vi "RT9031prueba.vi"() -> ()   [LabVIEW 2020]
uses:
  <vilib>/Model Interface Toolkit/Model Interface Toolkit.lvclass
  <vilib>/Platform/TimedLoop/XDataNode/timing_clust.ctl
  <vilib>/Platform/TimedLoop/XDataNode/nitl_modes.ctl
  <vilib>/Platform/TimedLoop/XDataNode/wakeup.ctl
  <vilib>/Model Interface Toolkit/Model Interface Toolkit.lvclass/Model Interface Toolkit.ctl
  <vilib>/Model Interface Toolkit/Model Update.vi
  <vilib>/Model Interface Toolkit/Tick Model.vi
  <vilib>/Model Interface Toolkit/Probe Signals.vi
  <vilib>/Model Interface Toolkit/Multirate/Dispatch Model Tasks.vi
  <vilib>/Model Interface Toolkit/Call Model Start Routine.vi
  <vilib>/Model Interface Toolkit/Handle Error.vi
  <vilib>/Model Interface Toolkit/Multirate/Wait on Tasks.vi
  <vilib>/FPGAPlugInAG/cRIO-9031/niLvFpga_Open_cRIO-9031.vi
  <vilib>/rvi/interface/common/dynamic/niFpgaDynamicAddResources.vi
  <vilib>/Utility/error.llb/Error Cluster From Error Code.vi
  <vilib>/rvi/errors/niLvFpgaAdjustHostInterfaceError.vi
  <vilib>/Model Interface Toolkit/Check Error.vi
  <vilib>/Model Interface Toolkit/Generate Error Cluster.vi
  <vilib>/Platform/TimedLoop/scheduler/LVUserAPI/Fire Software-Triggered Timing Source.vi
  <vilib>/FPGAPlugInAG/Dynamic/niLvFpga_Close_Dynamic.vi
  <vilib>/Platform/TimedLoop/XDataNode/XDataNode.xnode
  <vilib>/rvi/interface/nirviOpenFPGA/nirviOpenFPGA.xnode
  FPGA Bitfiles/dqmhemuladordege_FPGATarget_MainFPGA_ARUjFlg7-es.lvbitx
  FPGA/Main FPGA.vi
  <vilib>/rvi/interface/nirviReadWriteControl/nirviReadWriteControl.xnode
  <vilib>/rvi/interface/nirviCloseFPGA/nirviCloseFPGA.xnode
  <vilib>/Platform/TimedLoop/XDataNode/XDNodeRunTimeDep.lvlib
  NiFpgaLv.dll
  <vilib>/rvi/interface/Simulation/niFpgaSimulationCallBeginRW.vi
panel:
  in  "IFPGA 2":dbl
  in  "SOC 2":dbl
  in  "Igen 2":dbl
  in  "Vbat 2":dbl
  in  "Vgen 2":dbl
  in  "debug":bool
  out "FPGA":refnum<k20>
  out "SOC inicial [HMI]":dbl
  out "T. Bateria [HMI]":dbl
  out "I Load [HMI]":dbl
  out "Iexc":dbl(graph)
  out "Relé encendido":bool
  in  "Debug Iexc":bool
  in  "Iexc [Debug]":dbl
  in  "Modulacion Corrientes [Debug]":dbl
  in  "Debug Corrientes":bool
  in  "Modulacion T001 y T002 [Debug]":dbl
  in  "Debug Voltajes":bool
  out "stop!":i16
  out "0, 1":i16
  out "Estado de Carga":dbl(graph)
  out "Corriente Generador":dbl(graph)
  out "Voltaje Generador":dbl(graph)
  in  "wm(rpm)":dbl=1500.0
  out "Falla W4":bool
  out "Falla W3":bool
  out "Falla W2":bool
  out "Falla W1":bool
  out "Falla U4":bool
  out "Falla U3":bool
  out "Falla U2":bool
  out "Falla U1":bool
  out "Falla T002":bool
  out "Falla T001":bool
  out "Propulsion":bool
  out "CLC":bool
  out "ON/OFF":bool
  out "IFPGA":dbl
  out "Simulation Time (s)":dbl
  out "Iteration Duration":i64
  out "error out 2":errorcluster
  out "error out":errorcluster
  out "Finished Late? [i-1]":bool
  in  "stop FPGA":bool
  out "ExcFPGA":fxp<+/-,20,5>
  out "Igen":dbl
  out "Tbat":dbl
  out "IBat":dbl
  out "SOC":dbl
  out "Vbat":dbl
  out "Vgen":dbl
  out "Error2":errorcluster
  out "Model2":refnum<class "Model Interface Toolkit.lvclass">
  out "Error":errorcluster
  out "Model":refnum<class "Model Interface Toolkit.lvclass">
  in  "Relaunch Model/FPGA":bool
  in  "Prepare to Stop execution":bool
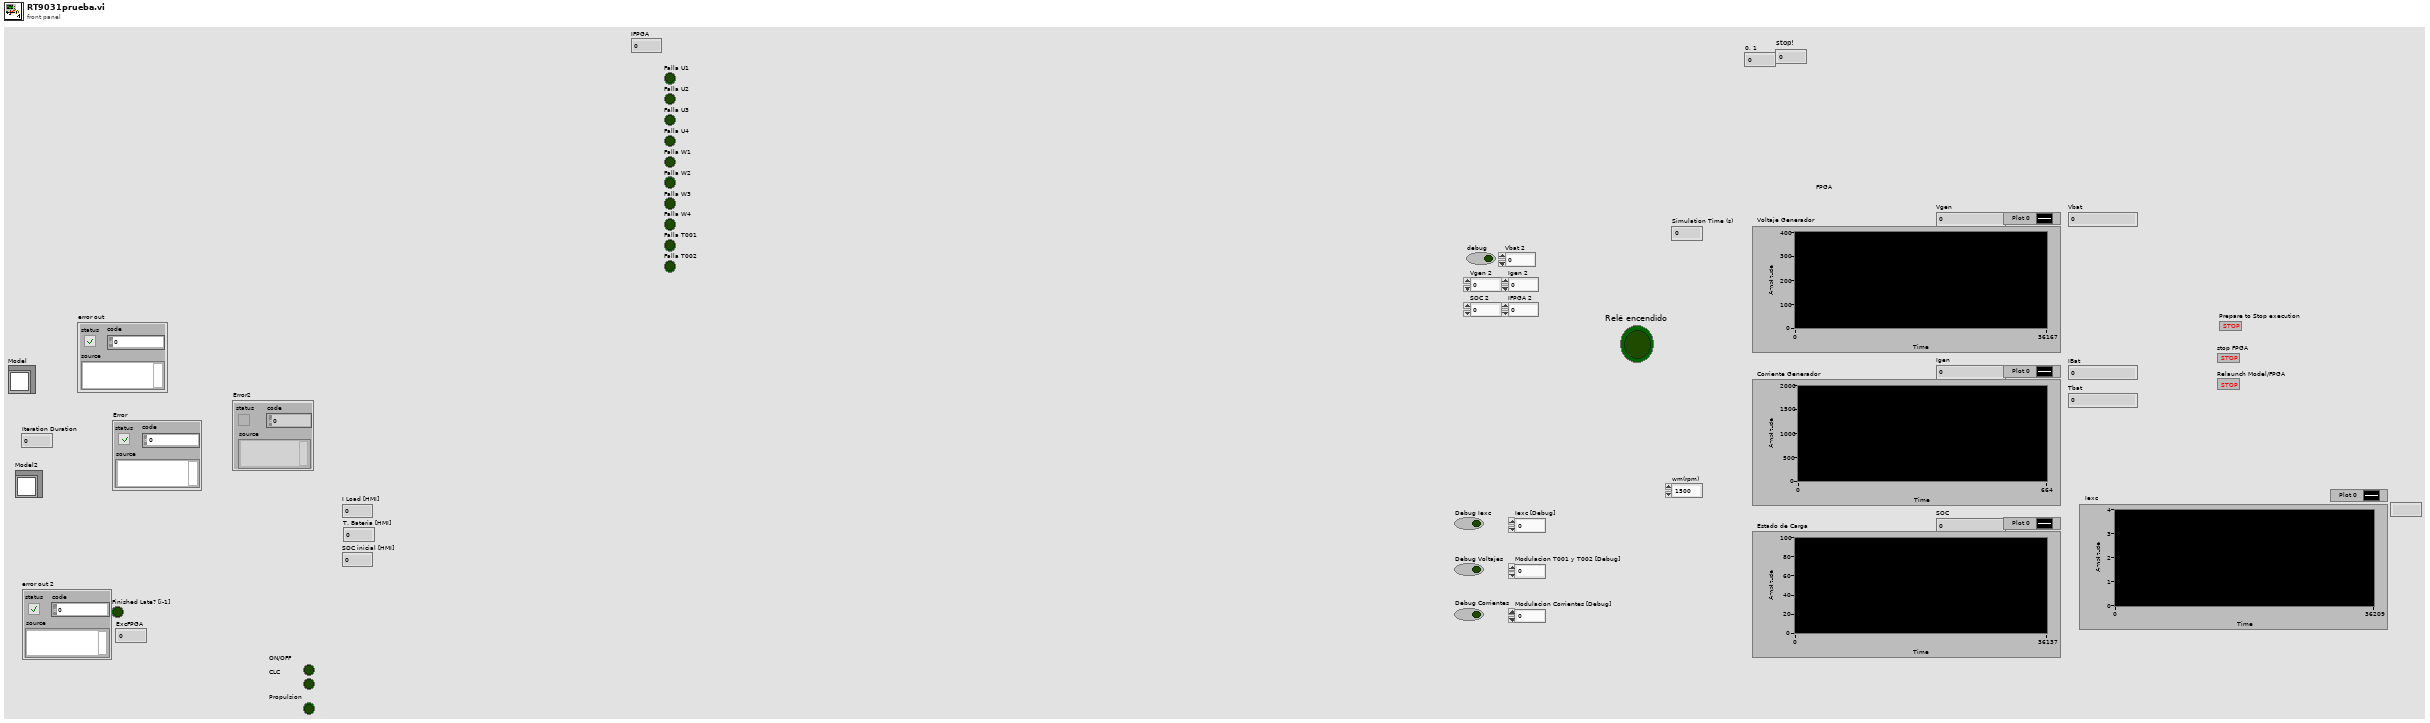
[diagram p1: front panel]
types:
  T1 = typedef "XDNodeRunTimeDep.lvlib/timing_clust.ctl" = cluster{"Expected End [f-1]":u64, "Actual End [f-1]":u64, "Finished Late? [f-1]":bool, "Expected End [i-1]":u64, "Actual End [i-1]":u64, "Finished Late? [i-1]":bool, "Expected Start [i]":u64, "Actual Start [i]":u64, "Expected Start [f]":u64, "Actual Start [f]":u64, "Source Name":string, "Structure Name":string, "Period":i64, "Deadline":i64, "Offset":i64, "Start":i64, "Priority":i32, "Timeout":i32, "Mode":T2, "Wakeup Reason":T3, "Error":errorcluster, "Source Type":string, "Secondary Source Type":string, "Global End Time":u64, "Global Start Time":u64, "Frame Duration":u64, "Iteration Duration":u64, "Assigned CPU":i32, "I/O Scan Engine Mode":u32}
  T2 = typedef "XDNodeRunTimeDep.lvlib/nitl_modes.ctl" = enum32{"No Change", "Process missed periods, maintain original phase", "Discard missed periods, maintain original phase", "Process missed periods, ignore original phase", "Discard missed periods, ignore original phase"}
  T3 = typedef "XDNodeRunTimeDep.lvlib/wakeup.ctl" = enum32{"Normal", "Aborted", "Asynchronous wakeup", "Timing source error", "Timed loop error", "Timeout"}
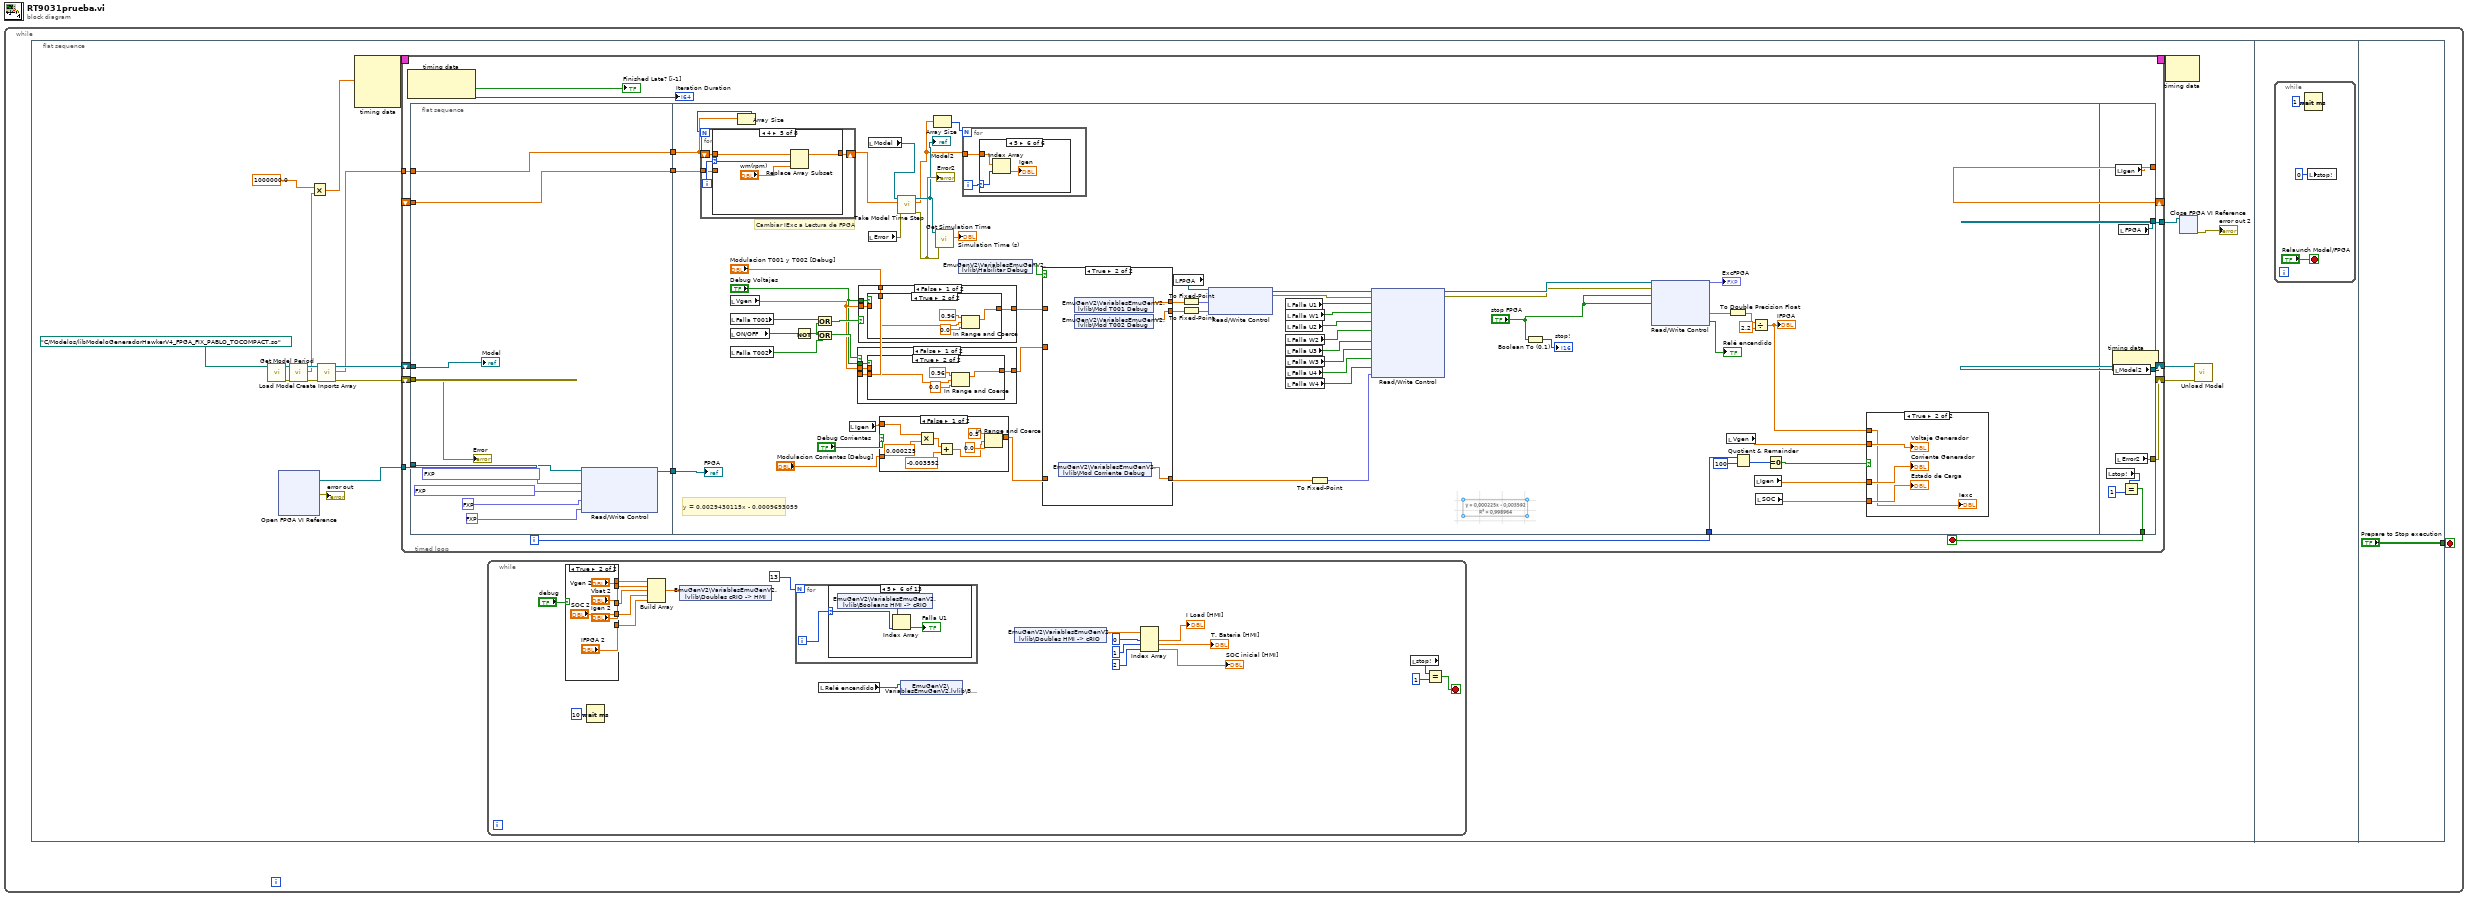
[diagram p0: block diagram]
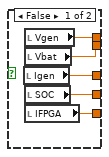
[diagram p2: hidden frame]
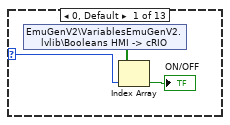
[diagram p3: hidden frame]
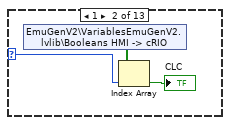
[diagram p4: hidden frame]
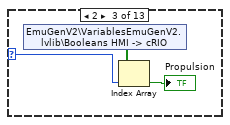
[diagram p5: hidden frame]
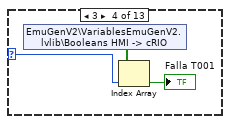
[diagram p6: hidden frame]
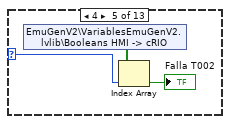
[diagram p7: hidden frame]
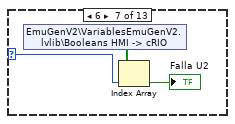
[diagram p8: hidden frame]
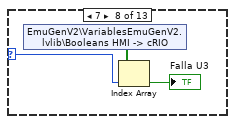
[diagram p9: hidden frame]
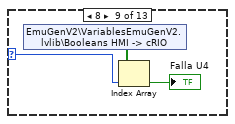
[diagram p10: hidden frame]
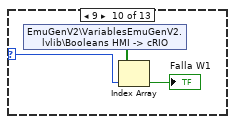
[diagram p11: hidden frame]
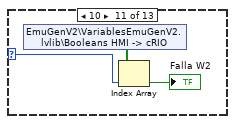
[diagram p12: hidden frame]
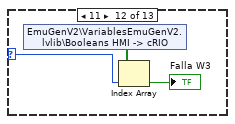
[diagram p13: hidden frame]
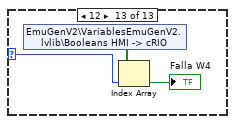
[diagram p14: hidden frame]
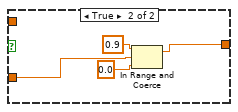
[diagram p16: hidden frame]
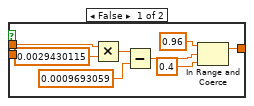
[diagram p17: hidden frame]
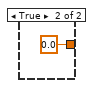
[diagram p18: hidden frame]
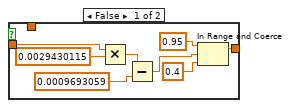
[diagram p19: hidden frame]
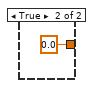
[diagram p20: hidden frame]
diagram:
  n1 = while {
    stop <- w1 stop-if-true
    n2 = flat-sequence {
      tunnel: ["Prepare to Stop execution"] -> w1
      frame #0 {
        n3 = call <vilib>:"Load Model.vi"("Model Path"=path "C:/Modelos/libModeloGeneradorHawkerV4_FPGA_FIX_PABLO_TOCOMPACT.so") -> ("error out"=w11:errorcluster, "Model out"=w10:refnum<class "Model Interface Toolkit.lvclass">)  [unwired: 9 in]
        n4 = xnode "Open FPGA VI Reference"() -> ("FPGA VI Reference Out"=w12:refnum<k20>, "error out"=→"error out":errorcluster)  [unwired: 2 in]
        n5 = call <vilib>:"Get Model Period.vi"("error in"=w11, "Model in"=w10) -> ("error out"=w9:errorcluster, "Model Period (s)"=w5:dbl, "Model out"=w7:refnum<class "Model Interface Toolkit.lvclass">)  [unwired: 7 in]
        n6 = Multiply(x=1000000.0, y=w5) -> (x*y=w6:dbl)
        n7 = call <vilib>:"Create Inports Array.vi"("error in (no error)"=w9, "Model in"=w7) -> ("error out"=w15:errorcluster, "Inports Array out"=w14:dbl[], "Model out"=w18:refnum<class "Model Interface Toolkit.lvclass">)  [unwired: 6 in, 1 out]
        n8 = node-c288(w6) -> (w20:T1)  [unwired: 3 in]
        n9 = timed-loop {
          timing: w20 -> [_]
          timing-out: [_] -> w19
          shift-right: [w101] -> w17
          shift-left: w18 -> [w106]
          shift-right: [w104] -> w16
          shift-left: w15 -> [w105]
          tunnel: w14 -> [w103]
          tunnel: [w100] -> w3
          tunnel: w12 -> [w97]
          shift-right: [w94] -> _
          shift-left: _ -> [w92]
          i -> [w91]
          stop <- w99 stop-if-true
          n10 = node-c288() -> (→"Finished Late? [i-1]":bool, →"Iteration Duration":i64)  [unwired: 1 in]
          n11 = flat-sequence {
            tunnel: w106 -> [w116]
            tunnel: w105 -> [w115]
            tunnel: w103 -> [w114]
            tunnel: [w114] -> w102
            tunnel: w97 -> [w112]
            tunnel: [w111] -> w96
            tunnel: [w113] -> w93
            tunnel: w92 -> [w113]
            tunnel: w102 -> [w177]
            tunnel: w96 -> [w129]
            tunnel: w93 -> [w174]
            tunnel: w91 -> [w164]
            tunnel: [w307] -> w101
            tunnel: [w306] -> w104
            tunnel: [w305] -> w100
            tunnel: [w304] -> w99
            tunnel: [w303] -> w94
            frame #0 {
              n12 = xnode "Read/Write Control"("FPGA VI Reference In"=w112, "Freq. PWM Volt."=fxp<+,32,0> 0.0005749999545514584, "Freq PWM Corr."=fxp<+,32,0> 0.0007249999325722456, "Fase PWM voltajes"=fxp<+,32,0> 0.0, "Fase PWM Corrientes"=fxp<+,32,0> 0.0) -> ("FPGA VI Reference Out"=w111:refnum<k20>)  [unwired: 1 in, 1 out]
              "Model" <- w116
              "Error" <- w115
            }
            frame #1 {
              # "y = 0,0029430115x - 0,0009693059"
              # "Cambiar IExc a Lectura de FPGA"
              n13 = local read "Vgen"() -> (w142:dbl)
              n14 = local read "Falla T001"() -> (w145:bool)
              n15 = local read "ON/OFF"() -> (w131:bool)
              n16 = local read "Falla T002"() -> (w146:bool)
              n17 = Array Size(array=w177) -> (size(s)=w176:i32)
              n18 = for {
                N: w176 -> [_]
                shift-right: [w255] -> w151
                shift-left: w177 -> [w256]
                tunnel: w174 -> [w254]
                i -> [w257]
                n19 = case shown="4" w257 {
                  selector: w257 -> [w261 w266 w269 w276 w282 w287 w290 w296]
                  tunnel: w256 -> [w262 w265 w270 w277 w283 w288 w293 w298]
                  tunnel: [w260 w264 w268 w275 w281 w286 w292 w297] -> w255
                  tunnel: w254 -> [_ _ _ _ _ _ _ _]
                  frame 0, Default {
                    n20 = local read "ON/OFF"() -> (w258:bool)
                    n21 = Boolean To (0,1)(Boolean=w258) -> (0, 1=w259:i16)
                    n22 = Replace Array Subset(array=w262, new element=w259, index=w261) -> (w260:dbl[])
                  }
                  frame 1 {
                    n23 = local read "I Load [HMI]"() -> (w263:dbl)
                    n24 = Replace Array Subset(array=w265, new element=w263, index=w266) -> (w264:dbl[])
                  }
                  frame 2 {
                    n25 = local read "SOC inicial [HMI]"() -> (w267:dbl)
                    n26 = Replace Array Subset(array=w270, new element=w267, index=w269) -> (w268:dbl[])
                  }
                  frame 3 {
                    n27 = local read "IFPGA"() -> (w273:dbl)
                    n28 = case shown="True" "Debug Iexc" {
                      tunnel: [w278 w279] -> w274
                      tunnel: w273 -> [w278 _]
                      tunnel: "Iexc [Debug]" -> [_ w279]
                      frame False {
                      }
                      frame True {
                      }
                    }
                    n29 = Replace Array Subset(array=w277, new element=w274, index=w276) -> (w275:dbl[])
                  }
                  frame 4 {
                    n30 = Replace Array Subset(array=w283, new element="wm(rpm)", index=w282) -> (w281:dbl[])
                  }
                  frame 5 {
                    n31 = local read "CLC"() -> (w284:bool)
                    n32 = Boolean To (0,1)(Boolean=w284) -> (0, 1=w285:i16)
                    n33 = Replace Array Subset(array=w288, new element=w285, index=w287) -> (w286:dbl[])
                  }
                  frame 6 {
                    n34 = local read "Propulsion"() -> (w289:bool)
                    n35 = Boolean To (0,1)(Boolean=w289) -> (0, 1=w291:i16)
                    "0, 1" <- w291
                    n36 = Replace Array Subset(array=w293, new element=w291, index=w290) -> (w292:dbl[])
                  }
                  frame 7 {
                    n37 = local read "0, 1"() -> (w295:i16)
                    n38 = case shown="1" w295 {
                      tunnel: [1 0] -> w294
                      frame 0, Default {
                      }
                      frame 1 {
                      }
                    }
                    n39 = Replace Array Subset(array=w298, new element=w294, index=w296) -> (w297:dbl[])
                  }
                }
              }
              n40 = Not(x=w131) -> (.not. x?=w147:bool)
              n41 = Or(x=w145, y=w147) -> (x .or. y?=w144:bool)
              n42 = Or(x=w147, y=w146) -> (x .or. y?=w143:bool)
              n43 = local read "Igen"() -> (w137:dbl)
              n44 = case shown="False" w143 {
                tunnel: w142 -> [w198 _]
                tunnel: [w199 0.0 ("upper limit")] -> w127
                tunnel: "Debug Voltajes" -> [w197 _]
                tunnel: "Modulacion T001 y T002 [Debug]" -> [w196 _]
                frame False {
                  n45 = case shown="True" w197 {
                    tunnel: [w205 w208] -> w199
                    tunnel: w198 -> [w204 _]
                    tunnel: w196 -> [_ w210]
                    frame False {
                      n46 = Multiply(x=w204, y=0.0029430115 ("bI Emulador")) -> (x*y=w202:dbl)
                      n47 = Subtract(x=w202, y=0.0009693059 ("mI Emulador")) -> (x-y=w200:dbl)
                      n48 = In Range and Coerce(upper limit=0.96, x=w200, lower limit=0.4) -> (coerced(x)=w205:dbl)  [unwired: 1 out]
                    }
                    frame True {
                      n49 = In Range and Coerce(upper limit=0.96, x=w210, lower limit=0.0) -> (coerced(x)=w208:dbl)  [unwired: 1 out]
                    }
                  }
                }
                frame True {
                }
              }
              n50 = case shown="False" w144 {
                tunnel: w142 -> [w215 _]
                tunnel: [w216 0.0 ("upper limit")] -> w125
                tunnel: "Debug Voltajes" -> [w214 _]
                tunnel: "Modulacion T001 y T002 [Debug]" -> [w213 _]
                frame False {
                  n51 = case shown="True" w214 {
                    tunnel: [w222 w225] -> w216
                    tunnel: w215 -> [w221 _]
                    tunnel: w213 -> [_ w227]
                    frame False {
                      n52 = Multiply(x=w221, y=0.0029430115 ("bI Emulador")) -> (x*y=w218:dbl)
                      n53 = Subtract(x=w218, y=0.0009693059 ("mI Emulador")) -> (x-y=w217:dbl)
                      n54 = In Range and Coerce(upper limit=0.95, x=w217, lower limit=0.4) -> (coerced(x)=w222:dbl)  [unwired: 1 out]
                    }
                    frame True {
                      n55 = In Range and Coerce(upper limit=0.96, x=w227, lower limit=0.0) -> (coerced(x)=w225:dbl)  [unwired: 1 out]
                    }
                  }
                }
                frame True {
                }
              }
              n56 = local read "Model"() -> (w152:refnum<class "Model Interface Toolkit.lvclass">)
              n57 = local read "Error"() -> (w153:errorcluster)
              n58 = case shown="False" "Debug Corrientes" {
                tunnel: [w189 w192] -> w121
                tunnel: w137 -> [w188 _]
                tunnel: "Modulacion Corrientes [Debug]" -> [_ w193]
                frame False {
                  n59 = Multiply(x=w188, y=0.000225) -> (x*y=w186:dbl)
                  n60 = Add(x=w186, y=-0.003592) -> (x+y=w184:dbl)
                  n61 = In Range and Coerce(upper limit=0.5, x=w184, lower limit=0.0) -> (coerced(x)=w189:dbl)  [unwired: 1 out]
                }
                frame True {
                  n62 = In Range and Coerce(upper limit=0.9, x=w193, lower limit=0.0) -> (coerced(x)=w192:dbl)  [unwired: 1 out]
                }
              }
              n63 = call <vilib>:"Take Model Time Step.vi"("error in (no error)"=w153, "Inport Array"=w151, "Model in"=w152) -> ("error out"=w150:errorcluster, "Outport Array out"=w148:dbl[], "Model out"=w149:refnum<class "Model Interface Toolkit.lvclass">)  [unwired: 6 in]
              "Model2" <- w149
              "Error2" <- w150
              n64 = Array Size(array=w148) -> (size(s)=w175:i32)
              n65 = call <vilib>:"Get Simulation Time.vi"("error in"=w150, "Model in"=w149) -> ("Simulation Time (s)"=→"Simulation Time (s)":dbl)  [unwired: 7 in, 2 out]
              n66 = shared-variable "EmuGenV2\\VariablesEmuGenV2.lvlib\\Habilitar Debug"() -> (w123:bool)  [unwired: 1 in, 1 out]
              n67 = for {
                N: w175 -> [_]
                tunnel: w148 -> [w234]
                i -> [w235]
                n68 = case shown="5" w235 {
                  selector: w235 -> [w237 w240 w243 w246 w249 w252]
                  tunnel: w234 -> [w238 w241 w244 w247 w250 w253]
                  frame 0, Default {
                    n69 = Index Array(array=w238, index=w237) -> (element=→"Vgen":dbl)
                  }
                  frame 1 {
                    n70 = Index Array(array=w241, index=w240) -> (element=→"Vbat":dbl)
                  }
                  frame 2 {
                    n71 = Index Array(array=w244, index=w243) -> (element=→"SOC":dbl)
                  }
                  frame 3 {
                    n72 = Index Array(array=w247, index=w246) -> (element=→"IBat":dbl)
                  }
                  frame 4 {
                    n73 = Index Array(array=w250, index=w249) -> (element=→"Tbat":dbl)
                  }
                  frame 5 {
                    n74 = Index Array(array=w253, index=w252) -> (element=→"Igen":dbl)
                  }
                }
              }
              n75 = case shown="True" w123 {
                tunnel: w127 -> [w180 _]
                tunnel: [w180 w182] -> w126
                tunnel: w125 -> [w179 _]
                tunnel: [w179 w183] -> w124
                tunnel: [w178 w181] -> w122
                tunnel: w121 -> [w178 _]
                frame False {
                }
                frame True {
                  n76 = shared-variable "EmuGenV2\\VariablesEmuGenV2.lvlib\\Mod Corriente Debug"() -> (w181:dbl)  [unwired: 1 in, 1 out]
                  n77 = shared-variable "EmuGenV2\\VariablesEmuGenV2.lvlib\\Mod T001 Debug"() -> (w183:dbl)  [unwired: 1 in, 1 out]
                  n78 = shared-variable "EmuGenV2\\VariablesEmuGenV2.lvlib\\Mod T002 Debug"() -> (w182:dbl)  [unwired: 1 in, 1 out]
                }
              }
              n79 = local read "FPGA"() -> (w128:refnum<k20>)
              n80 = To Fixed-Point(number=w124) -> (fixed-point=w119:fxp<+/-,16,1>)  [unwired: 1 in]
              n81 = To Fixed-Point(number=w126) -> (fixed-point=w118:fxp<+/-,16,1>)  [unwired: 1 in]
              n82 = xnode "Read/Write Control"("FPGA VI Reference In"=w128, "Modulacion T001"=w119, "Modulacion T002"=w118) -> ("FPGA VI Reference Out"=w163:refnum<k20>, "error out"=w154:errorcluster)  [unwired: 1 in]
              n83 = local read "Falla U1"() -> (w162:bool)
              n84 = local read "Falla W1"() -> (w161:bool)
              n85 = local read "Falla U2"() -> (w160:bool)
              n86 = local read "Falla W2"() -> (w159:bool)
              n87 = local read "Falla U3"() -> (w158:bool)
              n88 = local read "Falla W3"() -> (w157:bool)
              n89 = local read "Falla U4"() -> (w156:bool)
              n90 = local read "Falla W4"() -> (w155:bool)
              n91 = To Fixed-Point(number=w122) -> (fixed-point=w117:fxp<+,32,0>)  [unwired: 1 in]
              n92 = xnode "Read/Write Control"("FPGA VI Reference In"=w163, "error in"=w154, "Falla U1"=w162, "Falla W1"=w161, "Falla U2"=w160, "Falla W2"=w159, "Falla U3"=w158, "Falla W3"=w157, "Falla U4"=w156, "Falla W4"=w155, "Amplitud Corrientes"=w117) -> ("FPGA VI Reference Out"=w140:refnum<k20>, "error out"=w139:errorcluster)
              n93 = Boolean To (0,1)(Boolean="stop FPGA") -> (0, 1=→"stop!":i16)
              n94 = xnode "Read/Write Control"("FPGA VI Reference In"=w140, "error in"=w139, "Stop While"="stop FPGA", "STOP SCTL"="stop FPGA") -> ("IExc"=w138:fxp<+/-,20,5>, "Relé encendido"=→"Relé encendido":bool)  [unwired: 2 out]
              "ExcFPGA" <- w138
              n95 = local read "Vgen"() -> (w167:dbl)
              n96 = To Double Precision Float(number=w138) -> (double precision float=w172:dbl)
              n97 = Quotient & Remainder(x=w164, y=100) -> (x-y*floor(x/y)=w169:i32)  [unwired: 1 out]
              n98 = Divide(x=w172, y=2.2) -> (x/y=w132:dbl)
              "IFPGA" <- w132
              n99 = local read "Igen"() -> (w166:dbl)
              n100 = local read "SOC"() -> (w165:dbl)
              n101 = Equal To 0?(x=w169) -> (x = 0?=w168:bool)
              n102 = case shown="True" w168 {
                tunnel: w167 -> [_ w233]
                tunnel: w166 -> [_ w232]
                tunnel: w165 -> [_ w231]
                tunnel: w132 -> [_ w230]
                frame False {
                }
                frame True {
                  "Voltaje Generador" <- w233
                  "Corriente Generador" <- w232
                  "Estado de Carga" <- w231
                  "Iexc" <- w230
                }
              }
              "FPGA" <- w129
            }
            frame #2 {
              n103 = local read "stop!"() -> (w302:i16)
              n104 = local read "Model2"() -> (w307:refnum<class "Model Interface Toolkit.lvclass">)
              n105 = local read "Igen"() -> (w303:dbl)
              n106 = local read "Error2"() -> (w306:errorcluster)
              n107 = local read "FPGA"() -> (w305:refnum<k20>)
              n108 = Equal?(x=w302, y=i16 1) -> (x = y?=w304:bool)
            }
          }
          n109 = node-c288() -> ()  [unwired: 1 in, 1 out]
        }
        n110 = while {
          stop <- w40 stop-if-true
          n111 = case shown="True" "debug" {
            tunnel: [w45 "Vgen 2"] -> w39
            tunnel: [w44 "Vbat 2"] -> w38
            tunnel: [w43 "Igen 2"] -> w35
            tunnel: [w42 "SOC 2"] -> w32
            tunnel: [w41 "IFPGA 2"] -> w31
            frame False {
              n112 = local read "Igen"() -> (w43:dbl)
              n113 = local read "Vgen"() -> (w45:dbl)
              n114 = local read "Vbat"() -> (w44:dbl)
              n115 = local read "SOC"() -> (w42:dbl)
              n116 = local read "IFPGA"() -> (w41:dbl)
            }
            frame True {
            }
          }
          n117 = Wait (ms)(milliseconds to wait=u32 10) -> ()  [unwired: 1 out]
          n118 = Build Array(w39, w38, w35, w32, w31) -> (w37:dbl[])
          n119 = shared-variable "EmuGenV2\\VariablesEmuGenV2.lvlib\\Doubles cRIO -> HMI"(w37) -> ()  [unwired: 1 in, 1 out]
          n120 = for {
            N: 13 -> [_]
            i -> [w51]
            n121 = case shown="5" w51 {
              selector: w51 -> [w53 w56 w59 w62 w65 w68 w71 w74 w77 w80 w83 w86 w89]
              frame 0, Default {
                n122 = shared-variable "EmuGenV2\\VariablesEmuGenV2.lvlib\\Booleans HMI -> cRIO"() -> (w54:bool[])  [unwired: 1 in, 1 out]
                n123 = Index Array(array=w54, index=w53) -> (element=→"ON/OFF":bool)
              }
              frame 1 {
                n124 = shared-variable "EmuGenV2\\VariablesEmuGenV2.lvlib\\Booleans HMI -> cRIO"() -> (w57:bool[])  [unwired: 1 in, 1 out]
                n125 = Index Array(array=w57, index=w56) -> (element=→"CLC":bool)
              }
              frame 2 {
                n126 = shared-variable "EmuGenV2\\VariablesEmuGenV2.lvlib\\Booleans HMI -> cRIO"() -> (w60:bool[])  [unwired: 1 in, 1 out]
                n127 = Index Array(array=w60, index=w59) -> (element=→"Propulsion":bool)
              }
              frame 3 {
                n128 = shared-variable "EmuGenV2\\VariablesEmuGenV2.lvlib\\Booleans HMI -> cRIO"() -> (w63:bool[])  [unwired: 1 in, 1 out]
                n129 = Index Array(array=w63, index=w62) -> (element=→"Falla T001":bool)
              }
              frame 4 {
                n130 = shared-variable "EmuGenV2\\VariablesEmuGenV2.lvlib\\Booleans HMI -> cRIO"() -> (w66:bool[])  [unwired: 1 in, 1 out]
                n131 = Index Array(array=w66, index=w65) -> (element=→"Falla T002":bool)
              }
              frame 5 {
                n132 = shared-variable "EmuGenV2\\VariablesEmuGenV2.lvlib\\Booleans HMI -> cRIO"() -> (w69:bool[])  [unwired: 1 in, 1 out]
                n133 = Index Array(array=w69, index=w68) -> (element=→"Falla U1":bool)
              }
              frame 6 {
                n134 = shared-variable "EmuGenV2\\VariablesEmuGenV2.lvlib\\Booleans HMI -> cRIO"() -> (w72:bool[])  [unwired: 1 in, 1 out]
                n135 = Index Array(array=w72, index=w71) -> (element=→"Falla U2":bool)
              }
              frame 7 {
                n136 = shared-variable "EmuGenV2\\VariablesEmuGenV2.lvlib\\Booleans HMI -> cRIO"() -> (w75:bool[])  [unwired: 1 in, 1 out]
                n137 = Index Array(array=w75, index=w74) -> (element=→"Falla U3":bool)
              }
              frame 8 {
                n138 = shared-variable "EmuGenV2\\VariablesEmuGenV2.lvlib\\Booleans HMI -> cRIO"() -> (w78:bool[])  [unwired: 1 in, 1 out]
                n139 = Index Array(array=w78, index=w77) -> (element=→"Falla U4":bool)
              }
              frame 9 {
                n140 = shared-variable "EmuGenV2\\VariablesEmuGenV2.lvlib\\Booleans HMI -> cRIO"() -> (w81:bool[])  [unwired: 1 in, 1 out]
                n141 = Index Array(array=w81, index=w80) -> (element=→"Falla W1":bool)
              }
              frame 10 {
                n142 = shared-variable "EmuGenV2\\VariablesEmuGenV2.lvlib\\Booleans HMI -> cRIO"() -> (w84:bool[])  [unwired: 1 in, 1 out]
                n143 = Index Array(array=w84, index=w83) -> (element=→"Falla W2":bool)
              }
              frame 11 {
                n144 = shared-variable "EmuGenV2\\VariablesEmuGenV2.lvlib\\Booleans HMI -> cRIO"() -> (w87:bool[])  [unwired: 1 in, 1 out]
                n145 = Index Array(array=w87, index=w86) -> (element=→"Falla W3":bool)
              }
              frame 12 {
                n146 = shared-variable "EmuGenV2\\VariablesEmuGenV2.lvlib\\Booleans HMI -> cRIO"() -> (w90:bool[])  [unwired: 1 in, 1 out]
                n147 = Index Array(array=w90, index=w89) -> (element=→"Falla W4":bool)
              }
            }
          }
          n148 = local read "Relé encendido"() -> (w21:bool)
          n149 = shared-variable "EmuGenV2\\VariablesEmuGenV2.lvlib\\BUS DC ON"(w21) -> ()  [unwired: 1 in, 1 out]
          n150 = shared-variable "EmuGenV2\\VariablesEmuGenV2.lvlib\\Doubles HMI -> cRIO"() -> (w30:dbl[])  [unwired: 1 in, 1 out]
          n151 = Index Array(array=w30, index #1=0 ("index"), index #2=1 ("index"), index #3=2 ("index")) -> (element #1=→"I Load [HMI]":dbl, element #2=→"T. Bateria [HMI]":dbl, element #3=→"SOC inicial [HMI]":dbl)
          n152 = local read "stop!"() -> (w34:i16)
          n153 = Equal?(x=w34, y=i16 1) -> (x = y?=w40:bool)
        }
        n154 = node-c288(w19) -> ()  [unwired: 1 out]
        n155 = xnode "Close FPGA VI Reference"("FPGA VI Reference In"=w3) -> ("error out"=→"error out 2":errorcluster)  [unwired: 1 in]
        n156 = call <vilib>:"Unload Model.vi"("error in (no error)"=w16, "Model in"=w17) -> ()  [unwired: 9 in, 1 out]
      }
      frame #1 {
        n157 = while {
          stop <- "Relaunch Model/FPGA" stop-if-true
          n158 = Wait (ms)(milliseconds to wait=u32 1) -> ()  [unwired: 1 out]
          n159 = local write "stop!"(i16 0 ("stop!")) -> ()
        }
      }
      frame #2 {
      }
    }
  }
